vi "Overlay Edge Rake.vi"(4 "Edge Point Colors":u32(colorbox)=6618880, 6 "Rake Line Color":u32(colorbox)=16711680, 8 "error in":errorcluster, 9 "Search Lines":T2[](array[typedef]) {"Edge Info"."Distance (Real-World)" format="%.2f"; "Edge Info"."Location (Real-World)"."Y" format="%.2g"; "Edge Info"."Location (Real-World)"."X" format="%.2f"; "Edge Info"."Noise" format="%.2f"; "Edge Info"."Location (Pixel)"."Y" format="%.2g"; "Edge Info"."Location (Pixel)"."X" format="%.2f"; "Edge Info"."Strength" format="%.2f"; "Edge Info"."Distance (Pixel)" format="%.2f"}, 10 "Edges":T3[](array[typedef]) {"Distance (Real-World)" format="%.2f"; "Location (Real-World)"."Y" format="%.2g"; "Location (Real-World)"."X" format="%.2f"; "Noise" format="%.2f"; "Location (Pixel)"."Y" format="%.2g"; "Location (Pixel)"."X" format="%.2f"; "Strength" format="%.2f"; "Distance (Pixel)" format="%.2f"}, 11 "Image in":T1) -> (0 "error out":errorcluster, 3 "Image out":T1)   [LabVIEW 2013]
uses:
  <vilib>/vision/Measure.llb/Edge New.ctl
  <vilib>/vision/Image Controls.llb/IMAQ Image.ctl
  <vilib>/vision/Measure.llb/Search Line.ctl
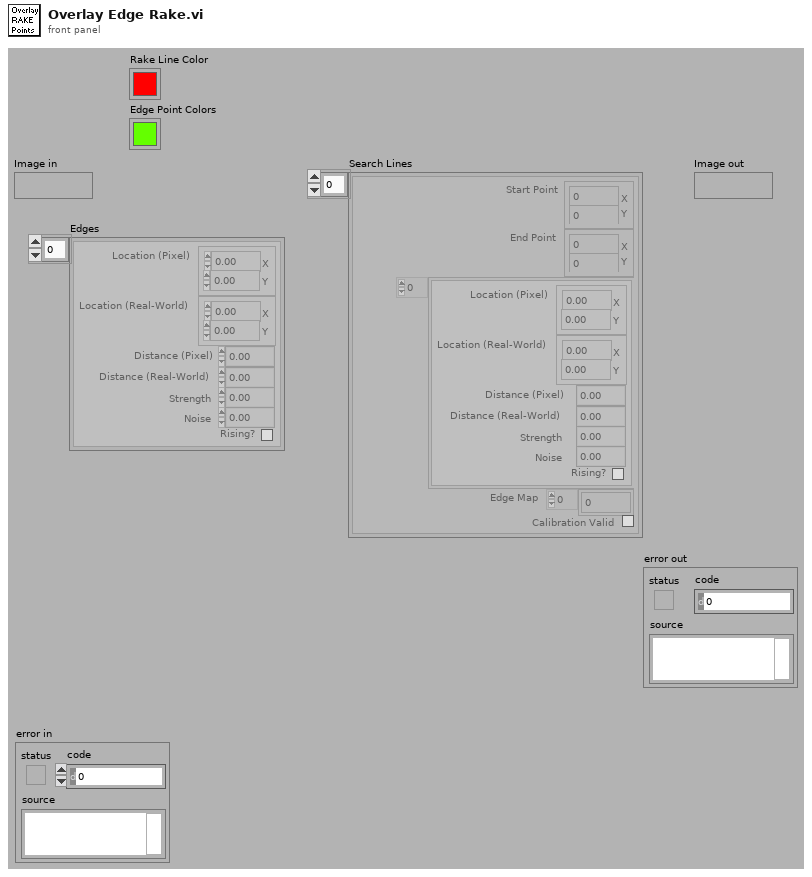
[diagram p1: front panel]
types:
  T1 = typedef "IMAQ Image.ctl" = refnum<image>
  T2 = typedef "Search Line.ctl" = cluster{"Start Point":cluster{"X":sgl, "Y":sgl}, "End Point":cluster{"X":sgl, "Y":sgl}, "Edge Info":T3[], "Edge Map":dbl[], "Calibration Valid":bool}
  T3 = typedef "Edge New.ctl" = cluster{"Location (Pixel)":cluster{"X":sgl, "Y":sgl}, "Location (Real-World)":cluster{"X":sgl, "Y":sgl}, "Distance (Pixel)":dbl, "Distance (Real-World)":dbl, "Strength":dbl, "Noise":dbl, "Rising?":bool}
  T4 = cluster{"Left":i32, "Top":i32, "Right":i32, "Bottom":i32}
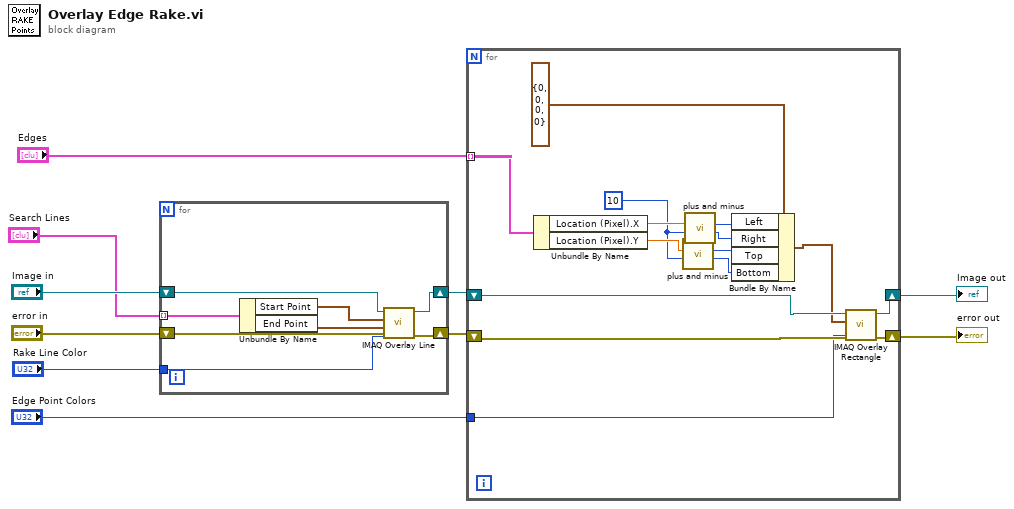
[diagram p0: block diagram]
diagram:
  n1 = for {
    shift-right: [w17] -> w7
    shift-left: "error in" -> [w18]
    tunnel: "Search Lines" -> [w14] mode=indexing
    shift-right: [w15] -> w6
    shift-left: "Image in" -> [w16]
    tunnel: "Rake Line Color" -> [w11]
    n2 = Unbundle By Name(w14) -> ("Start Point"=w13:cluster{"X":sgl, "Y":sgl}, "End Point"=w12:cluster{"X":sgl, "Y":sgl})
    n3 = call "IMAQ Overlay Line"("Color"=w11, "error in (no error)"=w18, "End Point"=w12, "Start Point"=w13, "Image"=w16) -> ("error out"=w17:errorcluster, "Image Out"=w15:T1)  [unwired: 1 in, 4 out]
  }
  n4 = for {
    shift-right: [w33] -> w2
    shift-left: w7 -> [w32]
    shift-right: [w31] -> w3
    shift-left: w6 -> [w29]
    tunnel: "Edges" -> [w20] mode=indexing
    tunnel: "Edge Point Colors" -> [w19]
    w21 = 10 ("b")
    n5 = Unbundle By Name(w20) -> ("Location (Pixel).X"=w27:sgl, "Location (Pixel).Y"=w24:sgl)
    n6 = call "plus and minus.vi"("b"=w21, "a"=w24) -> ("a-b"=w22:i32, "a+b"=w23:i32)  [unwired: 8 out]
    n7 = call "plus and minus.vi"("b"=w21, "a"=w27) -> ("a-b"=w25:i32, "a+b"=w26:i32)  [unwired: 8 out]
    n8 = Bundle By Name(cluster=T4 {"Left"=0, "Top"=0, "Right"=0, "Bottom"=0} ("Rectangle"), "Left"=w26, "Right"=w25, "Top"=w23, "Bottom"=w22) -> (w28:T4)
    n9 = call "IMAQ Overlay Rectangle"("Color"=w19, "error in (no error)"=w32, "Rectangle"=w28, "Image"=w29) -> ("error out"=w33:errorcluster, "Image Out"=w31:T1)  [unwired: 2 in, 4 out]
  }
  "Image out" <- w3
  "error out" <- w2
